vi "Camera parameter is gettable on fly.vi"(0 "AllCameraParameters":T1[](array[typedef]), 5 "Name":string) -> (4 "Gettable?":bool)   [LabVIEW 2020]
uses:
  Controls/ParameterID.ctl
  Controls/CameraParameters_Type.ctl
  Controls/CameraParameters_Authorization.ctl
  Controls/CameraParameters_OnFlyAuthorization.ctl
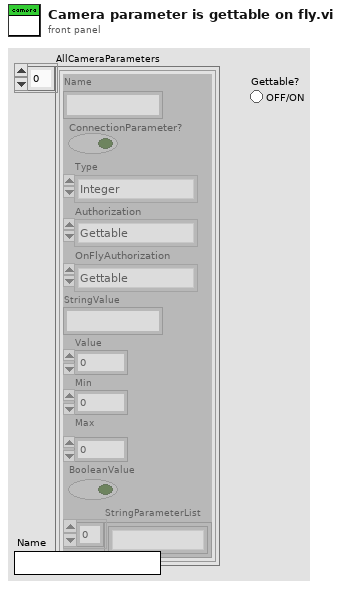
[diagram p1: front panel]
types:
  T1 = typedef "ParameterID.ctl" = cluster{"Name":string, "ConnectionParameter?":bool, "Type":T2, "Authorization":T3, "OnFlyAuthorization":T4, "StringValue":string, "Value":dbl, "Min":dbl, "Max":dbl, "BooleanValue":bool, "StringParameterList":string[]}
  T2 = typedef "CameraParameters_Type.ctl" = enum16{"Integer", "Real", "String", "Boolean"}
  T3 = typedef "CameraParameters_Authorization.ctl" = enum16{"Disable", "Gettable", "Settable - Gettable"}
  T4 = typedef "CameraParameters_OnFlyAuthorization.ctl" = enum16{"None", "Gettable", "Settable", "Settable - Gettable"}
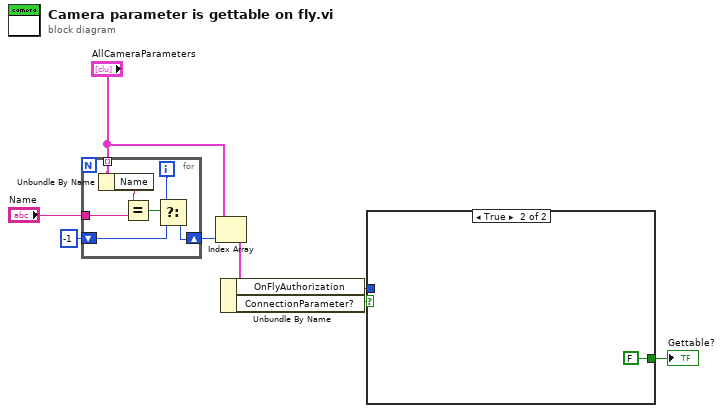
[diagram p0: block diagram]
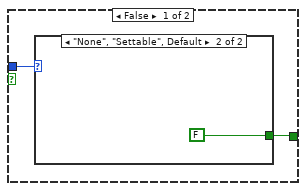
[diagram p2: hidden frame]
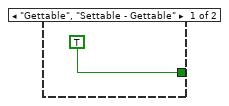
[diagram p3: hidden frame]
diagram:
  n1 = for {
    shift-right: [w13] -> w5
    shift-left: -1 -> [w12]
    tunnel: "AllCameraParameters" -> [w11] mode=indexing
    tunnel: "Name" -> [w9]
    i -> [w14]
    n2 = Unbundle By Name(w11) -> ("Name"=w10:string)
    n3 = Equal?(x=w10, y=w9) -> (x = y?=w15:bool)
    n4 = Select(t=w14, s=w15, f=w12) -> (s? t:f=w13:i32)
  }
  n5 = Index Array(array="AllCameraParameters", index=w5) -> (element=w7:T1)
  n6 = Unbundle By Name(w7) -> ("OnFlyAuthorization"=w3:T4, "ConnectionParameter?"=w1:bool)
  n7 = case shown="True" w1 {
    tunnel: w3 -> [w17 _]
    tunnel: [w16 FALSE] -> w2
    frame False {
      n8 = case shown="\"None\", \"Settable\", Default" w17 {
        tunnel: [TRUE FALSE] -> w16
        frame "Gettable", "Settable - Gettable" {
        }
        frame "None", "Settable", Default {
        }
      }
    }
    frame True {
    }
  }
  "Gettable?" <- w2
